vi "Programming.String.Count Number of Lines in a MultiLine String.vi"(4 "MultiLine String Input":string) -> (1 "Number of Lines":i32)   [LabVIEW 2010]
doc: "This VI determines the number of lines in a multi-line input\n\n\nChristopher G. Relf\ncrelf@viengineering.com"
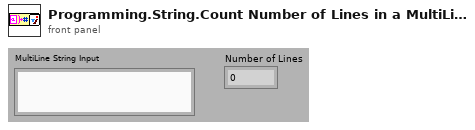
[diagram p1: front panel]
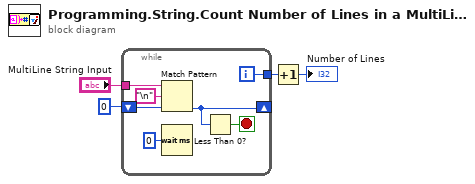
[diagram p0: block diagram]
diagram:
  n1 = while {
    tunnel: "MultiLine String Input" -> [w11]
    shift-right: [w7] -> _
    shift-left: 0 ("offset past match") -> [w10]
    tunnel: [w8] -> w2
    i -> [w8]
    stop <- w9 stop-if-true
    n2 = Match Pattern(string=w11, regular expression="\n", offset (0)=w10) -> (offset past match=w7:i32)  [unwired: 3 out]
    n3 = Wait (ms)(milliseconds to wait=u32 0) -> ()  [unwired: 1 out]
    n4 = Less Than 0?(x=w7) -> (x < 0?=w9:bool)
  }
  n5 = Increment(x=w2) -> (x+1=→"Number of Lines":i32)
